vi "Flatten To String.vi"(8 "error in (no error)":errorcluster, 10 "Variant":variant, 11 "JSON Serializer in":refnum<class "JSON Serializer.lvclass">) -> (0 "error out":errorcluster, 2 "String":string, 3 "JSON Serializer out":refnum<class "JSON Serializer.lvclass">)   [LabVIEW 2020, in "JKI JSON Serialization.lvlib" / "JSON Serializer.lvclass"]
doc: "Converts <b>Variant</b> to JSON formatted <b>String</b>."
uses:
  JSON Serializer.lvclass
  JSON Serializer.lvclass/JSON Serializer.ctl
  Library/Waveform Cluster.ctl
  <vilib>/Utility/error.llb/whitespace.ctl
  <userlib>/_OpenG.lib/lvdata/lvdata.llb/Get Collection Subtype__ogtk.vi
  <userlib>/_OpenG.lib/lvdata/lvdata.llb/openg_variant.lvlib
  <vilib>/Utility/VariantDataType/VariantType.lvlib
  JKI JSON Serialization.lvlib
  <vilib>/Utility/Data Type/NI_Data Type.lvlib
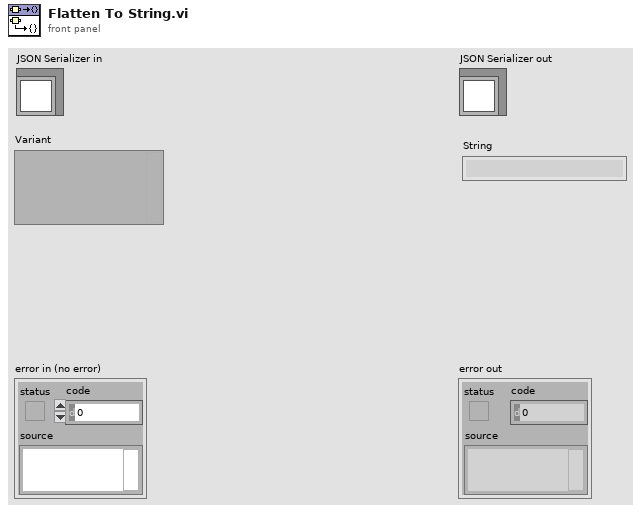
[diagram p1: front panel]
types:
  T1 = typedef "JKI JSON Serialization.lvlib/Waveform Cluster.ctl" = cluster{"t0":timestamp, "dt":dbl, "y":dbl[]}
  T2 = typedef "NI_Data Type.lvlib/Data Type.ctl" = enum8{"Invalid Type", "Void", "I8", "I16", "I32", "I64", "U8", "U16", "U32", "U64", "Single Float", "Double Float", "Extended Float", "Single Complex", "Double Complex", "Extended Complex", "Enum U8", "Enum U16", "Enum U32", "Enum U64", "Single Float With Unit", "Double Float With Unit", "Extended Float With Unit", "Single Complex with Unit", "Double Complex with Unit", "Extended Complex with Unit", "Boolean", "String", "Path", "Picture", "Tag", "Array", "Cluster", "Variant", "LV Variant", "Waveform", "Timestamp", "Digital Waveform", "Digital Data", "ExpressData", "Refnum", "External Data", "VI", "Poly VI", "LabVIEW Class Instance", "Fixed Point", "Set Collection", "Map Collection"}
  T3 = typedef "whitespace.ctl" = u16
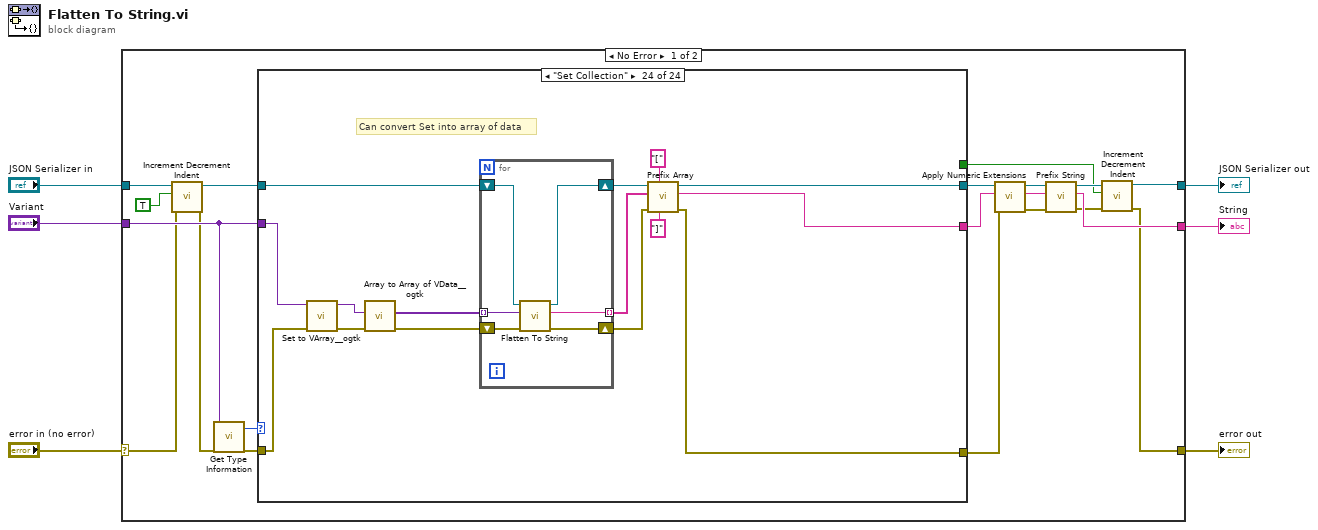
[diagram p0: block diagram]
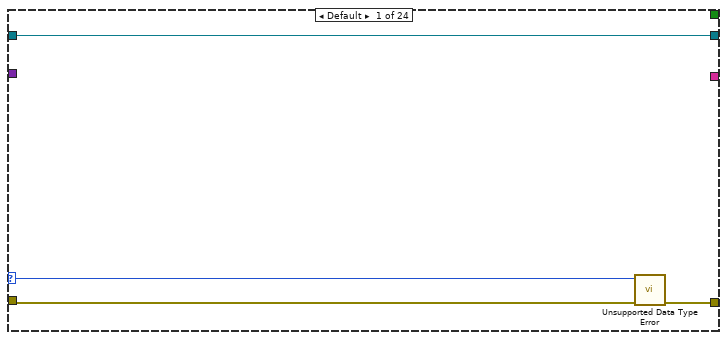
[diagram p2: hidden frame]
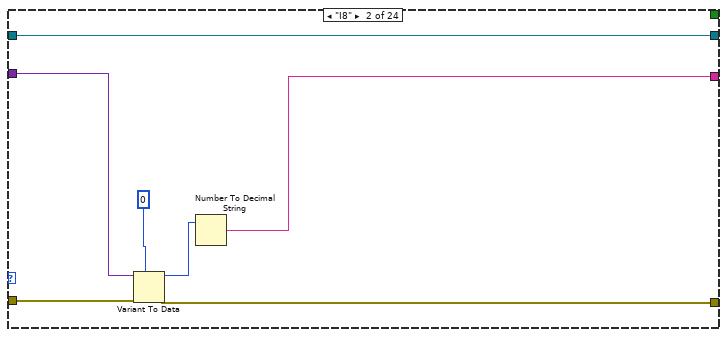
[diagram p3: hidden frame]
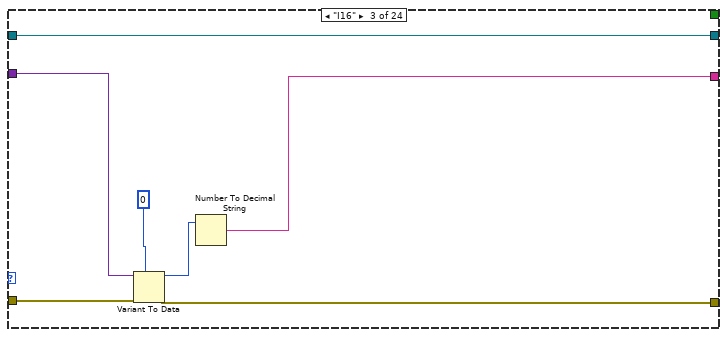
[diagram p4: hidden frame]
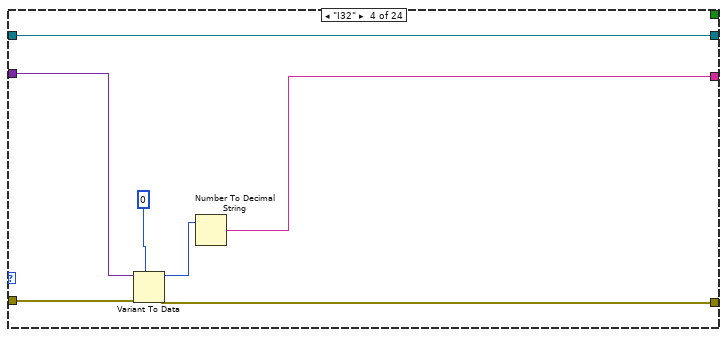
[diagram p5: hidden frame]
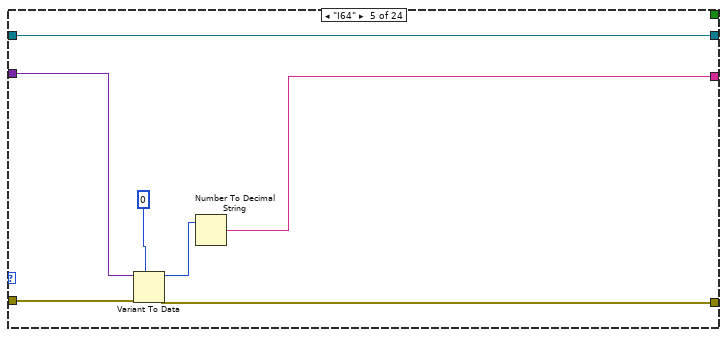
[diagram p6: hidden frame]
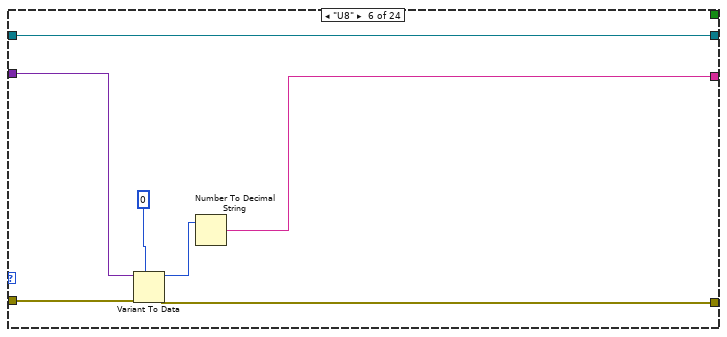
[diagram p7: hidden frame]
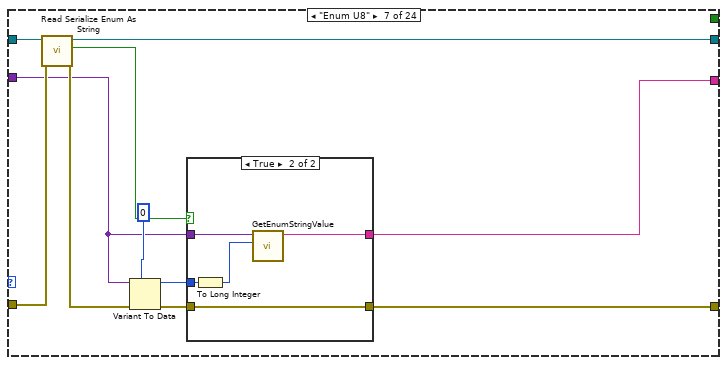
[diagram p8: hidden frame]
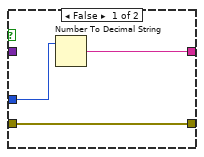
[diagram p9: hidden frame]
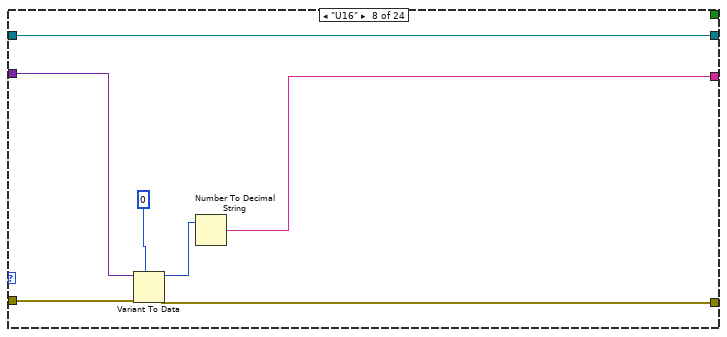
[diagram p10: hidden frame]
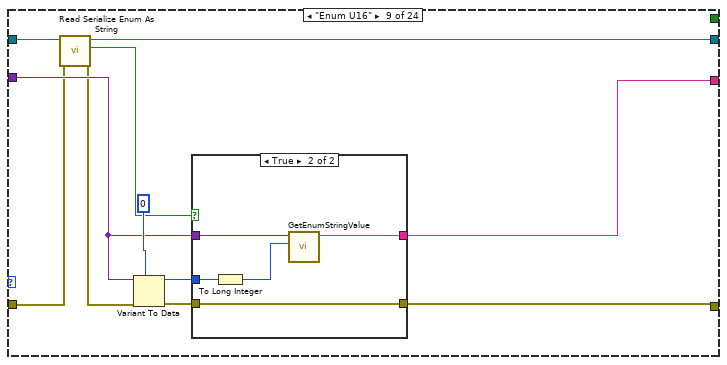
[diagram p11: hidden frame]
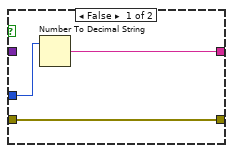
[diagram p12: hidden frame]
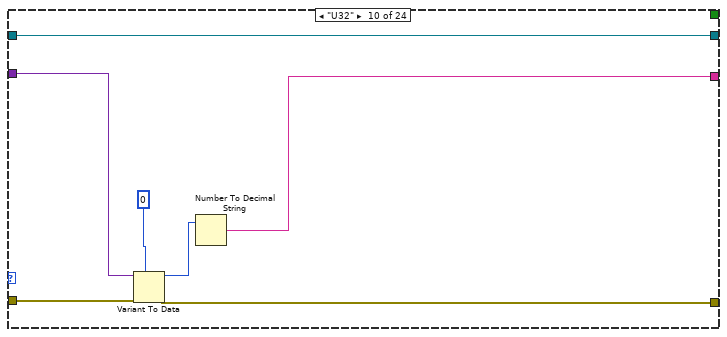
[diagram p13: hidden frame]
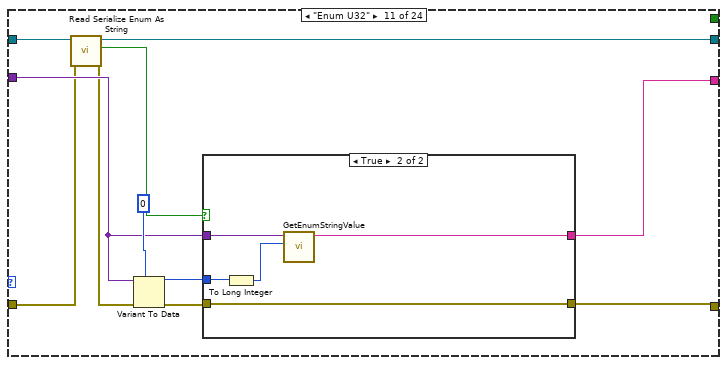
[diagram p14: hidden frame]
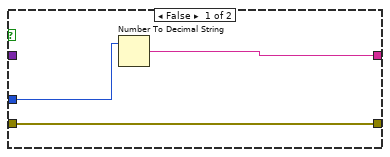
[diagram p15: hidden frame]
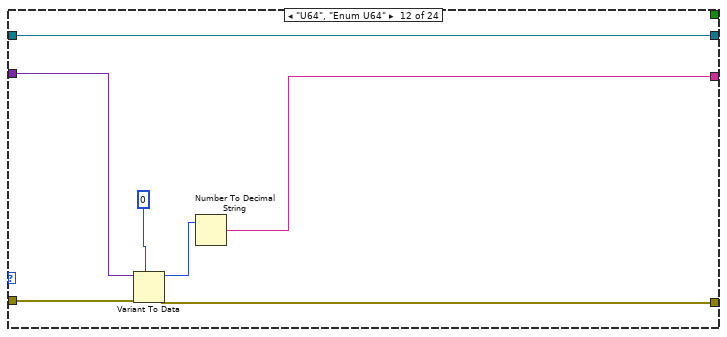
[diagram p16: hidden frame]
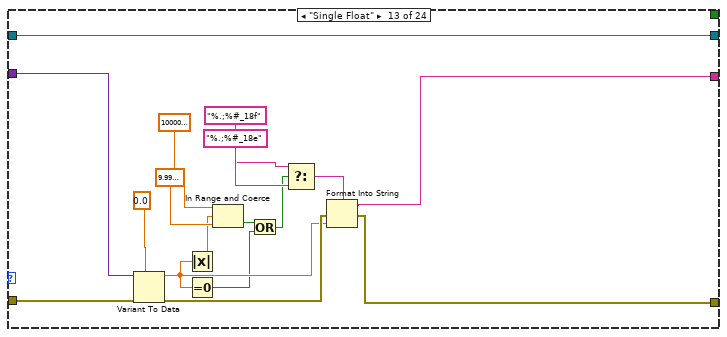
[diagram p17: hidden frame]
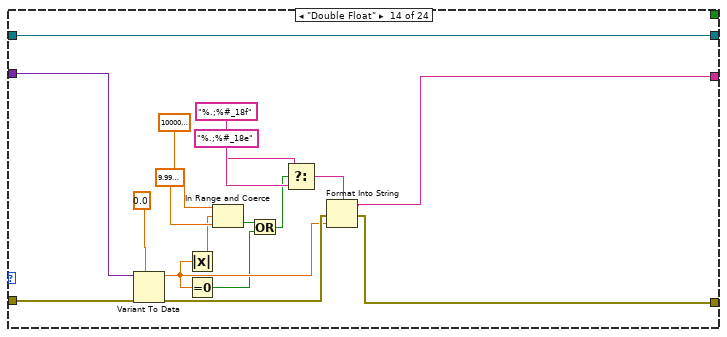
[diagram p18: hidden frame]
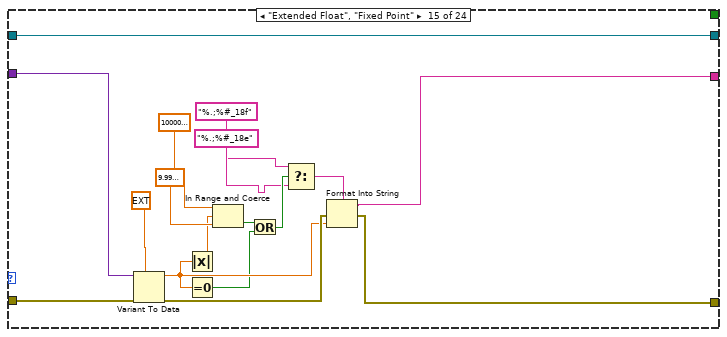
[diagram p19: hidden frame]
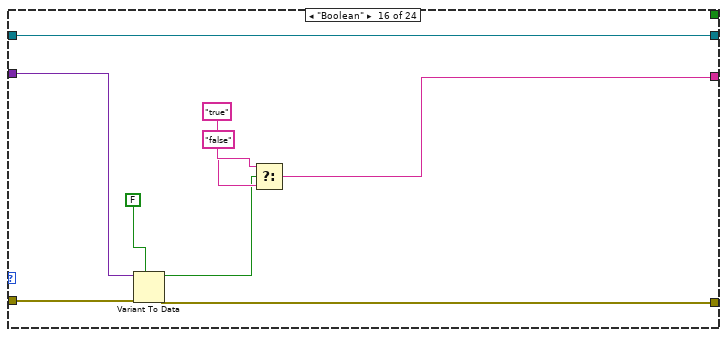
[diagram p20: hidden frame]
diagram:
  n1 = case shown="No Error" "error in (no error)" {
    selector: "error in (no error)" -> [w19 w466]
    tunnel: [w8 w466] -> w5
    tunnel: [w10 w465] -> w3
    tunnel: "JSON Serializer in" -> [w21 w465]
    tunnel: "Variant" -> [w24 _]
    tunnel: [w13 _] -> w1
    frame No Error {
      n2 = call "Increment Decrement Indent.vi"("error in (no error)"=w19, "Increment"=TRUE, "JSON Serializer in"=w21) -> ("error out"=w18:errorcluster, "JSON Serializer out"=w20:refnum<class "JSON Serializer.lvclass">)  [unwired: 7 in]
      n3 = call <vilib>:"Get Type Information.vi"("error in (no error)"=w18, "variant"=w24) -> ("error out"=w25:errorcluster, "type"=w26:T2)  [unwired: 5 in, 3 out]
      n4 = case shown="\"Set Collection\"" w26 {
        selector: w26 -> [w27 _ _ _ _ _ _ _ _ _ _ _ _ _ _ _ w204 w251 _ _ _ _ _ _]
        tunnel: w20 -> [w30 w37 w44 w51 w58 w65 w75 w91 w96 w117 w126 w143 w160 w177 w194 w203 w209 w249 w281 w293 w342 w402 w429 w450]
        tunnel: [w30 w37 w44 w51 w58 w65 w74 w91 w95 w117 w125 w143 w160 w177 w194 w203 w209 w248 w280 w292 w345 w405 w425 w446] -> w16
        tunnel: [w29 w31 w38 w45 w52 w59 w66 w85 w99 w111 w123 w137 w155 w172 w189 w195 w206 w252 w270 w291 w344 w404 w423 w444] -> w23
        tunnel: w25 -> [w28 w36 w43 w50 w57 w64 w73 w90 w94 w116 w119 w142 w159 w176 w193 w202 w208 w250 w285 w288 w346 w401 w428 w449]
        tunnel: [_ w32 w39 w46 w53 w60 w76 w86 w98 w112 w124 w138 w151 w168 w186 w197 w205 w246 w269 w290 w343 w403 w424 w445] -> w22
        tunnel: w24 -> [_ w35 w42 w49 w56 w63 w68 w89 w97 w115 w120 w141 w158 w175 w192 w201 w207 w244 w284 w289 w347 w399 w437 w458]
        tunnel: [_ _ _ _ _ _ _ _ _ _ _ _ _ _ _ _ _ _ _ _ w337 _ _ _] -> w7
        frame Default {
          n5 = call "Unsupported Data Type Error.vi"("error in (no error)"=w28, "Type Enum"=w27) -> ("error out"=w29:errorcluster)  [unwired: 9 in]
        }
        frame "I8" {
          n6 = Variant To Data(error in=w36, type=i8 0, Variant=w35) -> (data=w33:i8, error out=w31:errorcluster)
          n7 = Number To Decimal String(number=w33) -> (decimal integer string=w32:string)  [unwired: 1 in]
        }
        frame "I16" {
          n8 = Variant To Data(error in=w43, type=i16 0, Variant=w42) -> (data=w40:i16, error out=w38:errorcluster)
          n9 = Number To Decimal String(number=w40) -> (decimal integer string=w39:string)  [unwired: 1 in]
        }
        frame "I32" {
          n10 = Variant To Data(error in=w50, type=0, Variant=w49) -> (data=w47:i32, error out=w45:errorcluster)
          n11 = Number To Decimal String(number=w47) -> (decimal integer string=w46:string)  [unwired: 1 in]
        }
        frame "I64" {
          n12 = Variant To Data(error in=w57, type=i64 0, Variant=w56) -> (data=w54:i64, error out=w52:errorcluster)
          n13 = Number To Decimal String(number=w54) -> (decimal integer string=w53:string)  [unwired: 1 in]
        }
        frame "U8" {
          n14 = Variant To Data(error in=w64, type=u8 0, Variant=w63) -> (data=w61:u8, error out=w59:errorcluster)
          n15 = Number To Decimal String(number=w61) -> (decimal integer string=w60:string)  [unwired: 1 in]
        }
        frame "Enum U8" {
          n16 = call-dynamic "Read Serialize Enum As String.vi"("error in (no error)"=w73, "JSON Serializer in"=w75) -> ("error out"=w72:errorcluster, "Enums As String?"=w69:bool, "JSON Serializer out"=w74:refnum<class "JSON Serializer.lvclass">)  [unwired: 7 in]
          n17 = Variant To Data(error in=w72, type=u8 0, Variant=w68) -> (data=w70:u8, error out=w67:errorcluster)
          n18 = case shown="True" w69 {
            tunnel: [w79 w80] -> w76
            tunnel: w70 -> [w78 w82]
            tunnel: w68 -> [_ w83]
            tunnel: w67 -> [w77 w84]
            tunnel: [w77 w84] -> w66
            frame False {
              n19 = Number To Decimal String(number=w78) -> (decimal integer string=w79:string)  [unwired: 1 in]
            }
            frame True {
              n20 = To Long Integer(number=w82) -> (32bit integer=w81:i32)
              n21 = call "GetEnumStringValue.vi"("Index"=w81, "Enum Variant"=w83) -> ("string"=w80:string)  [unwired: 9 in]
            }
          }
        }
        frame "U16" {
          n22 = Variant To Data(error in=w90, type=u16 0, Variant=w89) -> (data=w87:u16, error out=w85:errorcluster)
          n23 = Number To Decimal String(number=w87) -> (decimal integer string=w86:string)  [unwired: 1 in]
        }
        frame "Enum U16" {
          n24 = call-dynamic "Read Serialize Enum As String.vi"("error in (no error)"=w94, "JSON Serializer in"=w96) -> ("error out"=w93:errorcluster, "Enums As String?"=w92:bool, "JSON Serializer out"=w95:refnum<class "JSON Serializer.lvclass">)  [unwired: 7 in]
          n25 = Variant To Data(error in=w93, type=u16 0, Variant=w97) -> (data=w101:u16, error out=w100:errorcluster)
          n26 = case shown="True" w92 {
            tunnel: [w105 w106] -> w98
            tunnel: w101 -> [w104 w108]
            tunnel: w97 -> [_ w109]
            tunnel: w100 -> [w103 w107]
            tunnel: [w103 w107] -> w99
            frame False {
              n27 = Number To Decimal String(number=w104) -> (decimal integer string=w105:string)  [unwired: 1 in]
            }
            frame True {
              n28 = To Long Integer(number=w108) -> (32bit integer=w110:i32)
              n29 = call "GetEnumStringValue.vi"("Index"=w110, "Enum Variant"=w109) -> ("string"=w106:string)  [unwired: 9 in]
            }
          }
        }
        frame "U32" {
          n30 = Variant To Data(error in=w116, type=u32 0, Variant=w115) -> (data=w113:u32, error out=w111:errorcluster)
          n31 = Number To Decimal String(number=w113) -> (decimal integer string=w112:string)  [unwired: 1 in]
        }
        frame "Enum U32" {
          n32 = call-dynamic "Read Serialize Enum As String.vi"("error in (no error)"=w119, "JSON Serializer in"=w126) -> ("error out"=w118:errorcluster, "Enums As String?"=w127:bool, "JSON Serializer out"=w125:refnum<class "JSON Serializer.lvclass">)  [unwired: 7 in]
          n33 = Variant To Data(error in=w118, type=u32 0, Variant=w120) -> (data=w121:u32, error out=w122:errorcluster)
          n34 = case shown="True" w127 {
            tunnel: [w131 w132] -> w124
            tunnel: w121 -> [w130 w133]
            tunnel: w120 -> [_ w134]
            tunnel: w122 -> [w129 w136]
            tunnel: [w129 w136] -> w123
            frame False {
              n35 = Number To Decimal String(number=w130) -> (decimal integer string=w131:string)  [unwired: 1 in]
            }
            frame True {
              n36 = To Long Integer(number=w133) -> (32bit integer=w135:i32)
              n37 = call "GetEnumStringValue.vi"("Index"=w135, "Enum Variant"=w134) -> ("string"=w132:string)  [unwired: 9 in]
            }
          }
        }
        frame "U64", "Enum U64" {
          n38 = Variant To Data(error in=w142, type=u64 0, Variant=w141) -> (data=w139:u64, error out=w137:errorcluster)
          n39 = Number To Decimal String(number=w139) -> (decimal integer string=w138:string)  [unwired: 1 in]
        }
        frame "Single Float" {
          n40 = Variant To Data(error in=w159, type=sgl 0.0, Variant=w158) -> (data=w149:sgl, error out=w156:errorcluster)
          n41 = Absolute Value(x=w149) -> (abs(x)=w150:sgl)
          n42 = Equal To 0?(x=w149) -> (x = 0?=w148:bool)
          n43 = In Range and Coerce(upper limit=sgl 1000000.0, x=w150, lower limit=sgl 0.0001 ("upper limit")) -> (In Range?=w147:bool)  [unwired: 1 out]
          n44 = Or(x=w147, y=w148) -> (x .or. y?=w146:bool)
          n45 = Select(t="%.;%#_18f" ("format string"), s=w146, f="%.;%#_18e" ("format string")) -> (s? t:f=w144:string)
          n46 = Format Into String(format string=w144, error in=w156, w149) -> (resulting string=w151:string, error out=w155:errorcluster)  [unwired: 1 in]
        }
        frame "Double Float" {
          n47 = Variant To Data(error in=w176, type=0.0, Variant=w175) -> (data=w166:dbl, error out=w173:errorcluster)
          n48 = Absolute Value(x=w166) -> (abs(x)=w167:dbl)
          n49 = Equal To 0?(x=w166) -> (x = 0?=w165:bool)
          n50 = In Range and Coerce(upper limit=sgl 1000000.0, x=w167, lower limit=sgl 0.0001 ("upper limit")) -> (In Range?=w164:bool)  [unwired: 1 out]
          n51 = Or(x=w164, y=w165) -> (x .or. y?=w163:bool)
          n52 = Select(t="%.;%#_18f" ("format string"), s=w163, f="%.;%#_18e" ("format string")) -> (s? t:f=w161:string)
          n53 = Format Into String(format string=w161, error in=w173, w166) -> (resulting string=w168:string, error out=w172:errorcluster)  [unwired: 1 in]
        }
        frame "Extended Float", "Fixed Point" {
          n54 = Variant To Data(error in=w193, type=ext 0.0, Variant=w192) -> (data=w184:ext, error out=w190:errorcluster)
          n55 = Absolute Value(x=w184) -> (abs(x)=w185:ext)
          n56 = Equal To 0?(x=w184) -> (x = 0?=w183:bool)
          n57 = In Range and Coerce(upper limit=sgl 1000000.0, x=w185, lower limit=sgl 0.0001 ("upper limit")) -> (In Range?=w182:bool)  [unwired: 1 out]
          n58 = Or(x=w182, y=w183) -> (x .or. y?=w181:bool)
          n59 = Select(t="%.;%#_18f" ("format string"), s=w181, f="%.;%#_18e" ("format string")) -> (s? t:f=w178:string)
          n60 = Format Into String(format string=w178, error in=w190, w184) -> (resulting string=w186:string, error out=w189:errorcluster)  [unwired: 1 in]
        }
        frame "Boolean" {
          n61 = Variant To Data(error in=w202, type=FALSE, Variant=w201) -> (data=w196:bool, error out=w195:errorcluster)
          n62 = Select(t="true" ("format string"), s=w196, f="false" ("format string")) -> (s? t:f=w197:string)
        }
        frame "String", "Path" {
          n63 = case shown="\"Path\"" w204 {
            tunnel: w208 -> [w217 w243]
            tunnel: w207 -> [w216 w242]
            tunnel: [w215 w238] -> w206
            tunnel: [w214 w232] -> w205
            frame "Path" {
              n64 = Variant To Data(error in=w217, type=path "", Variant=w216) -> (data=w210:path, error out=w212:errorcluster)
              n65 = Not A Number/Path/Refnum?(number/path/refnum=w210) -> (NaN/Path/Refnum?=w211:bool)
              n66 = case shown="True" w211 {
                tunnel: [w226 w230] -> w215
                tunnel: [w220 "null" ("JSON string")] -> w214
                tunnel: w212 -> [w218 w230]
                tunnel: w210 -> [w219 _]
                frame False {
                  n67 = Path To String(path=w219) -> (string=w227:string)
                  n68 = Build Array(w227) -> (w228:string[])
                  n69 = Flatten To JSON(anything=w228, error in (no error)=w218) -> (JSON string=w224:string, 11:w226:errorcluster)  [unwired: 1 in]
                  n70 = String Length(string=w224) -> (length=w223:i32)
                  n71 = Subtract(x=w223, y=2) -> (x-y=w221:i32)
                  n72 = String Subset(string=w224, offset (0)=1, length (rest)=w221) -> (substring=w220:string)
                }
                frame True {
                }
              }
            }
            frame "String", Default {
              n73 = Variant To Data(error in=w243, type="", Variant=w242) -> (data=w240:string, error out=w239:errorcluster)
              n74 = Build Array(w240) -> (w241:string[])
              n75 = Flatten To JSON(anything=w241, error in (no error)=w239) -> (JSON string=w236:string, 11:w238:errorcluster)  [unwired: 1 in]
              n76 = String Length(string=w236) -> (length=w235:i32)
              n77 = Subtract(x=w235, y=2) -> (x-y=w233:i32)
              n78 = String Subset(string=w236, offset (0)=1, length (rest)=w233) -> (substring=w232:string)
            }
          }
        }
        frame "Timestamp" {
          n79 = Unbundle By Name(w249) -> ("timestamps"=w247:bool, "universal time"=w245:bool)
          n80 = case shown="True" w247 {
            tunnel: [w256 w257] -> w252
            tunnel: w251 -> [w255 _]
            tunnel: w250 -> [w254 w267]
            tunnel: w249 -> [w253 w268]
            tunnel: [w253 w268] -> w248
            tunnel: [_ w259] -> w246
            tunnel: w245 -> [_ w262]
            tunnel: w244 -> [_ w266]
            frame False {
              n81 = call "Unsupported Data Type Error.vi"("error in (no error)"=w254, "Type Enum"=w255) -> ("error out"=w256:errorcluster)  [unwired: 9 in]
            }
            frame True {
              n82 = Variant To Data(error in=w267, type=timestamp(0 s since 1904-01-01), Variant=w266) -> (data=w265:timestamp, error out=w263:errorcluster)
              n83 = call "Timestamp To ISO String.vi"("error in (no error)"=w263, "Universal time (F)"=w262, "Timestamp"=w265) -> ("error out"=w258:errorcluster, "ISO Timestamp String"=w260:string)  [unwired: 7 in]
              n84 = Format Into String(format string="\"%s\"", error in=w258, w260) -> (resulting string=w259:string, error out=w257:errorcluster)  [unwired: 1 in]
            }
          }
        }
        frame "Waveform" {
          n85 = call "Increment Decrement Indent.vi"("JSON Serializer in"=w281) -> ("JSON Serializer out"=w274:refnum<class "JSON Serializer.lvclass">)  [unwired: 9 in, 1 out]
          n86 = Variant To Data(error in=w285, type=waveform(dbl) {"t0"=timestamp(0 s since 1904-01-01), "dt"=1.0, "Y"=[]}, Variant=w284) -> (data=w279:waveform(dbl), error out=w271:errorcluster)
          n87 = Unbundle By Name(w279) -> ("t0"=w277:timestamp, "dt"=w276:dbl, "Y"=w275:dbl[])
          n88 = Bundle By Name(cluster=T1 {"t0"=timestamp(0 s since 1904-01-01), "dt"=1.0, "y"=[]} ("waveform"), "t0"=w277, "dt"=w276, "y"=w275) -> (w272:T1)
          n89 = call-dynamic "Flatten To String.vi"("error in (no error)"=w271, "Variant"=w272, "JSON Serializer in"=w274) -> ("error out"=w270:errorcluster, "String"=w269:string, "JSON Serializer out"=w273:refnum<class "JSON Serializer.lvclass">)  [unwired: 6 in]
          n90 = call "Increment Decrement Indent.vi"("Increment"=TRUE, "JSON Serializer in"=w273) -> ("JSON Serializer out"=w280:refnum<class "JSON Serializer.lvclass">)  [unwired: 8 in, 1 out]
        }
        frame "Array" {
          n91 = call <vilib>:"GetArrayInfo.vi"("error in (no error)"=w288, "Variant"=w289) -> ("error out"=w287:errorcluster, "NDims"=w286:i32)  [unwired: 6 in, 2 out]
          n92 = case shown="1" w286 {
            tunnel: w293 -> [w294 w310 w330]
            tunnel: [w294 w307 w329] -> w292
            tunnel: [w297 w305 w328] -> w291
            tunnel: [_ w304 w327] -> w290
            tunnel: w287 -> [w295 w300 w325]
            tunnel: w289 -> [_ w299 w326]
            frame 0, Default {
              n93 = call <vilib>:"Error Cluster From Error Code.vi"("error in (no error)"=w295, "error message (\"\")"="Flattening failed. Zero or negative dimensional arrays not supported." ("error message (\"\")"), "error code (0)"=1) -> ("error out"=w297:errorcluster)  [unwired: 6 in]
            }
            frame 1 {
              n94 = call <userlib>:"Array to Array of VData__ogtk.vi"("error in (no error)"=w300, "MultiD Array"=w299) -> ("error out"=w309:errorcluster, "1D Array of Variants"=w311:variant[])  [unwired: 8 in]
              n95 = for {
                tunnel: w311 -> [w317] mode=indexing
                shift-right: [w315] -> w308
                shift-left: w310 -> [w316]
                tunnel: [w314] -> w303 mode=indexing
                shift-right: [w313] -> w306
                shift-left: w309 -> [w312]
                n96 = call-dynamic "Flatten To String.vi"("error in (no error)"=w312, "Variant"=w317, "JSON Serializer in"=w316) -> ("error out"=w313:errorcluster, "String"=w314:string, "JSON Serializer out"=w315:refnum<class "JSON Serializer.lvclass">)  [unwired: 6 in]
              }
              n97 = call "Prefix Array.vi"("End Symbol"="]", "Start Symbol"="[", "error in (no error)"=w306, "Array"=w303, "JSON Serializer in"=w308) -> ("error out"=w305:errorcluster, "String"=w304:string, "JSON Serializer out"=w307:refnum<class "JSON Serializer.lvclass">)  [unwired: 4 in]
            }
            frame 2.. {
              n98 = call "MultiD Array to 1D Array of VArrays.vi"("error in (no error)"=w325, "MultiD Array"=w326) -> ("error out"=w324:errorcluster, "Array of VArrays"=w323:variant[])  [unwired: 8 in]
              n99 = for {
                tunnel: w323 -> [w336] mode=indexing
                shift-right: [w334] -> w322
                shift-left: w330 -> [w335]
                tunnel: [w333] -> w320 mode=indexing
                shift-right: [w332] -> w321
                shift-left: w324 -> [w331]
                n100 = call-dynamic "Flatten To String.vi"("error in (no error)"=w331, "Variant"=w336, "JSON Serializer in"=w335) -> ("error out"=w332:errorcluster, "String"=w333:string, "JSON Serializer out"=w334:refnum<class "JSON Serializer.lvclass">)  [unwired: 6 in]
              }
              n101 = call "Prefix Array.vi"("End Symbol"="]", "Start Symbol"="[", "error in (no error)"=w321, "Array"=w320, "JSON Serializer in"=w322) -> ("error out"=w328:errorcluster, "String"=w327:string, "JSON Serializer out"=w329:refnum<class "JSON Serializer.lvclass">)  [unwired: 4 in]
            }
          }
        }
        frame "Cluster" {
          n102 = call "Cluster Info.vi"("error in (no error)"=w346, "Cluster Variant"=w347) -> ("error out"=w341:errorcluster, "Name"=w338:string, "Treat As Array"=w339:bool, "Cluster Elements"=w340:variant[])  [unwired: 6 in]
          n103 = case shown="False" w339 {
            tunnel: [w358 w388] -> w345
            tunnel: [w356 w385] -> w344
            tunnel: [w352 w391] -> w343
            tunnel: w342 -> [w351 w390]
            tunnel: w341 -> [w349 w383]
            tunnel: w340 -> [w348 w395]
            tunnel: w338 -> [_ w394]
            tunnel: [_ w380] -> w337
            frame False {
              # "Treat cluster as an object"
              n104 = Unbundle By Name(w351) -> ("multiline?"=w350:bool)
              n105 = for {
                tunnel: w348 -> [w360] mode=indexing
                shift-right: [w370] -> w359
                shift-left: w351 -> [w375]
                tunnel: [w372] -> w353 mode=indexing
                shift-right: [w373] -> w357
                shift-left: w349 -> [w363]
                tunnel: w350 -> [w364]
                n106 = call "Variant Metadata.vi"("error in (no error)"=w363, "Variant"=w360) -> ("error out"=w362:errorcluster, "Name"=w361:string)  [unwired: 7 in, 1 out]
                n107 = call-dynamic "Flatten To String.vi"("error in (no error)"=w362, "Variant"=w360, "JSON Serializer in"=w375) -> ("error out"=w374:errorcluster, "String"=w366:string, "JSON Serializer out"=w371:refnum<class "JSON Serializer.lvclass">)  [unwired: 6 in]
                n108 = case shown="True" w364 {
                  tunnel: w366 -> [w376 w379]
                  tunnel: [w376 w377] -> w365
                  frame False {
                  }
                  frame True {
                    w378 = T3 1 items=["both", "start of string", "end of string"] ("location (both)")
                    n109 = call <vilib>:"Trim Whitespace.vi"("string"=w379, "location (both)"=w378) -> ("trimmed string"=w377:string)
                  }
                }
                n110 = call-dynamic "Flatten To String.vi"("error in (no error)"=w374, "Variant"=w361, "JSON Serializer in"=w371) -> ("error out"=w369:errorcluster, "String"=w368:string, "JSON Serializer out"=w370:refnum<class "JSON Serializer.lvclass">)  [unwired: 6 in]
                n111 = Format Into String(format string="%s:%s", error in=w369, w368, w365) -> (resulting string=w372:string, error out=w373:errorcluster)  [unwired: 1 in]
              }
              n112 = call "Prefix Array.vi"("End Symbol"="}", "Start Symbol"="{", "error in (no error)"=w357, "Array"=w353, "JSON Serializer in"=w359) -> ("error out"=w356:errorcluster, "String"=w352:string, "JSON Serializer out"=w358:refnum<class "JSON Serializer.lvclass">)  [unwired: 4 in]
            }
            frame True {
              # "https://github.com/JKISoftware/JKI-JSON-Serialization/issues/31"
              # "Fix for GitHub Issue 31\nIncorrect indentation when treating cluster as an ordered array"
              # "Treat cluster as an ordered array"
              n113 = call "Increment Decrement Indent.vi"("error in (no error)"=w383, "Increment"=FALSE, "JSON Serializer in"=w390) -> ("error out"=w382:errorcluster, "JSON Serializer out"=w389:refnum<class "JSON Serializer.lvclass">)  [unwired: 7 in]
              n114 = call <userlib>:"Set Data Name__ogtk.vi"("error in (no error)"=w382, "Data Name"=w394, "Data"=w395) -> ("error out"=w393:errorcluster, "Renamed Data"=w392:variant)  [unwired: 7 in]
              n115 = call-dynamic "Flatten To String.vi"("error in (no error)"=w393, "Variant"=w392, "JSON Serializer in"=w389) -> ("error out"=w386:errorcluster, "String"=w391:string, "JSON Serializer out"=w387:refnum<class "JSON Serializer.lvclass">)  [unwired: 6 in]
              n116 = flat-sequence {
                tunnel: [FALSE ("Increment")] -> w384
                tunnel: [TRUE ("Increment")] -> w380
                frame #0 {
                }
              }
              n117 = call "Increment Decrement Indent.vi"("error in (no error)"=w386, "Increment"=w384, "JSON Serializer in"=w387) -> ("error out"=w385:errorcluster, "JSON Serializer out"=w388:refnum<class "JSON Serializer.lvclass">)  [unwired: 7 in]
            }
          }
        }
        frame "LV Variant" {
          n118 = call "Null Value.vi"() -> ("Null"=w398:variant)
          n119 = Equal?(x=w399, y=w398) -> (x = y?=w400:bool)
          n120 = case shown="False" w400 {
            tunnel: [w419 w422] -> w405
            tunnel: [w418 w421] -> w404
            tunnel: [w417 "null" ("String")] -> w403
            tunnel: w402 -> [w416 w422]
            tunnel: w401 -> [w409 w421]
            tunnel: w399 -> [w406 _]
            frame False {
              n121 = call "Increment Decrement Indent.vi"("error in (no error)"=w409, "JSON Serializer in"=w416) -> ("error out"=w411:errorcluster, "JSON Serializer out"=w415:refnum<class "JSON Serializer.lvclass">)  [unwired: 8 in]
              n122 = Variant To Data(error in=w411, type=variant ("variant"), Variant=w406) -> (data=w408:variant, error out=w407:errorcluster)
              n123 = call-dynamic "Flatten To String.vi"("error in (no error)"=w407, "Variant"=w408, "JSON Serializer in"=w415) -> ("error out"=w413:errorcluster, "String"=w417:string, "JSON Serializer out"=w414:refnum<class "JSON Serializer.lvclass">)  [unwired: 6 in]
              n124 = call "Increment Decrement Indent.vi"("error in (no error)"=w413, "Increment"=TRUE, "JSON Serializer in"=w414) -> ("error out"=w418:errorcluster, "JSON Serializer out"=w419:refnum<class "JSON Serializer.lvclass">)  [unwired: 7 in]
            }
            frame True {
            }
          }
        }
        frame "Map Collection" {
          # "Can convert Map into array of key-value clusters"
          n125 = call <userlib>:"Map to VArray of Clusters__ogtk.vi"("error in"=w428, "Map"=w437) -> ("error out"=w427:errorcluster, "Array of Clusters (key-value)"=w431:variant)  [unwired: 8 in]
          n126 = call <userlib>:"Array to Array of VData__ogtk.vi"("error in (no error)"=w427, "MultiD Array"=w431) -> ("error out"=w426:errorcluster, "1D Array of Variants"=w430:variant[])  [unwired: 8 in]
          n127 = for {
            tunnel: w430 -> [w443] mode=indexing
            shift-right: [w441] -> w436
            shift-left: w429 -> [w442]
            tunnel: [w440] -> w434 mode=indexing
            shift-right: [w439] -> w435
            shift-left: w426 -> [w438]
            n128 = call-dynamic "Flatten To String.vi"("error in (no error)"=w438, "Variant"=w443, "JSON Serializer in"=w442) -> ("error out"=w439:errorcluster, "String"=w440:string, "JSON Serializer out"=w441:refnum<class "JSON Serializer.lvclass">)  [unwired: 6 in]
          }
          n129 = call "Prefix Array.vi"("End Symbol"="]", "Start Symbol"="[", "error in (no error)"=w435, "Array"=w434, "JSON Serializer in"=w436) -> ("error out"=w423:errorcluster, "String"=w424:string, "JSON Serializer out"=w425:refnum<class "JSON Serializer.lvclass">)  [unwired: 4 in]
        }
        frame "Set Collection" {
          # "Can convert Set into array of data"
          n130 = call <userlib>:"Set to VArray__ogtk.vi"("error in"=w449, "Set"=w458) -> ("error out"=w448:errorcluster, "Array"=w452:variant)  [unwired: 8 in]
          n131 = call <userlib>:"Array to Array of VData__ogtk.vi"("error in (no error)"=w448, "MultiD Array"=w452) -> ("error out"=w447:errorcluster, "1D Array of Variants"=w451:variant[])  [unwired: 8 in]
          n132 = for {
            tunnel: w451 -> [w464] mode=indexing
            shift-right: [w462] -> w457
            shift-left: w450 -> [w463]
            tunnel: [w461] -> w455 mode=indexing
            shift-right: [w460] -> w456
            shift-left: w447 -> [w459]
            n133 = call-dynamic "Flatten To String.vi"("error in (no error)"=w459, "Variant"=w464, "JSON Serializer in"=w463) -> ("error out"=w460:errorcluster, "String"=w461:string, "JSON Serializer out"=w462:refnum<class "JSON Serializer.lvclass">)  [unwired: 6 in]
          }
          n134 = call "Prefix Array.vi"("End Symbol"="]", "Start Symbol"="[", "error in (no error)"=w456, "Array"=w455, "JSON Serializer in"=w457) -> ("error out"=w444:errorcluster, "String"=w445:string, "JSON Serializer out"=w446:refnum<class "JSON Serializer.lvclass">)  [unwired: 4 in]
        }
      }
      n135 = call "Apply Numeric Extensions.vi"("error in (no error)"=w23, "JSON string in"=w22, "JSON Serializer in"=w16) -> ("error out"=w9:errorcluster, "JSON string out"=w14:string, "JSON Serializer out"=w15:refnum<class "JSON Serializer.lvclass">)  [unwired: 6 in]
      n136 = call "Prefix String.vi"("error in (no error)"=w9, "Input String"=w14, "JSON Serializer in"=w15) -> ("error out"=w11:errorcluster, "Output String"=w13:string, "JSON Serializer out"=w12:refnum<class "JSON Serializer.lvclass">)  [unwired: 6 in]
      n137 = call "Increment Decrement Indent.vi"("error in (no error)"=w11, "Increment"=w7, "JSON Serializer in"=w12) -> ("error out"=w8:errorcluster, "JSON Serializer out"=w10:refnum<class "JSON Serializer.lvclass">)  [unwired: 7 in]
    }
    frame Error {
    }
  }
  "error out" <- w5
  "JSON Serializer out" <- w3
  "String" <- w1
